vi "elliptsoid fitting.vi"(11 "data in":dbl[][](array[numeric])) -> (1 "b":dbl, 2 "n":dbl[](array[numeric]), 3 "M":T1)   [LabVIEW 2021]
uses:
  <vilib>/Analysis/Matrix/Datatypes/RealMatrix.ctl
  <vilib>/Analysis/7linalg.llb/Eigenvalue and Vectors Output Option.ctl
  <vilib>/Analysis/baseanly.llb/Real A x B.vi
  <vilib>/Analysis/_algsub.llb/Real PseudoInverse Matrix.vi
  <vilib>/Analysis/7linalg.llb/Real Transpose Matrix.vi
  <vilib>/Analysis/7linalg.llb/Real Generalized Eigenvalues and Vectors.vi
  <vilib>/Analysis/baseanly.llb/A x Vector.vi
  <vilib>/Analysis/Matrix/Numeric/Subtract/Subtract - RM,RM.vi
  <vilib>/Analysis/NI_AALBase.lvlib
  <vilib>/Analysis/NI_AALPro.lvlib
  <vilib>/Analysis/Matrix/NI_Matrix.lvlib
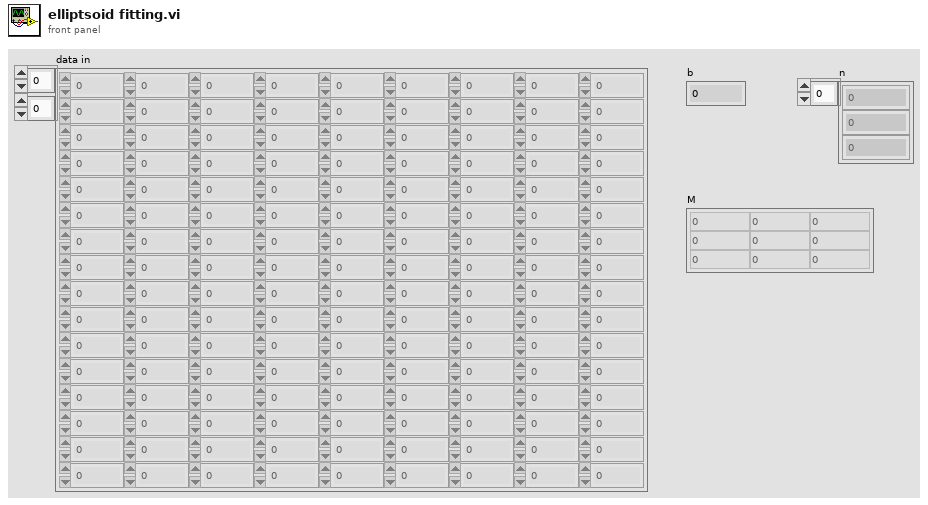
[diagram p1: front panel]
types:
  T1 = typedef "NI_Matrix.lvlib/RealMatrix.ctl" = dbl[][]
  T2 = typedef "NI_AALPro.lvlib/Eigenvalue and Vectors Output Option.ctl" = i32
  T3 = typedef "NI_Matrix.lvlib/ComplexMatrix.ctl" = cdb[][]
  T4 = cluster{"[0]":dbl, "[1]":dbl, "[2]":dbl, "[3]":dbl, "[4]":dbl, "[5]":dbl, "[6]":dbl, "[7]":dbl, "[8]":dbl, "[9]":dbl}
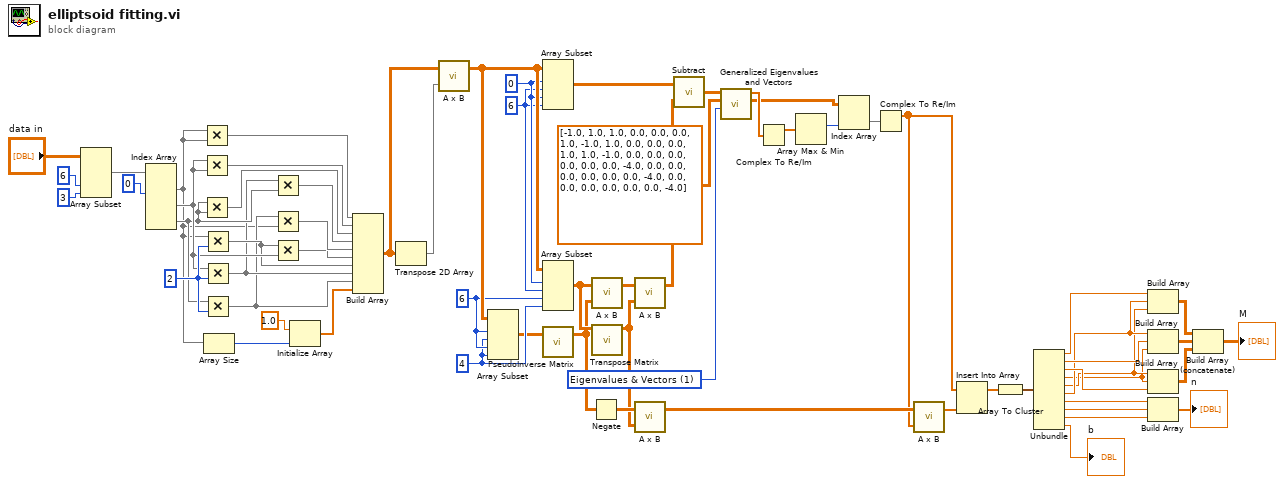
[diagram p0: block diagram]
diagram:
  w31 = T2 1 items=["Eigenvalues", "Eigenvalues & Vectors"] ("output option")
  w37 = 4 ("length")
  w38 = 6 ("index")
  w39 = 6 ("length")
  w40 = 0 ("index")
  w56 = 2 ("y")
  n1 = Array Subset(array="data in", index (col)=6 ("index"), length (col)=3 ("length")) -> (w61:dbl[][])  [unwired: 2 in]
  n2 = Index Array(array=w61, index (col) #1=0 ("disabled index (col)")) -> (element #1=w46:dbl[], element #2=w54:dbl[], element #3=w53:dbl[])  [unwired: 5 in]
  n3 = Multiply(x=w46, y=w46) -> (x*y=w59:dbl[])
  n4 = Multiply(x=w54, y=w54) -> (x*y=w58:dbl[])
  n5 = Multiply(x=w53, y=w53) -> (x*y=w57:dbl[])
  n6 = Multiply(x=w46, y=w56) -> (x*y=w50:dbl[])
  n7 = Multiply(x=w54, y=w56) -> (x*y=w49:dbl[])
  n8 = Multiply(x=w53, y=w56) -> (x*y=w48:dbl[])
  n9 = Array Size(array=w46) -> (size(s)=w45:i32)
  n10 = Multiply(x=w49, y=w53) -> (x*y=w55:dbl[])
  n11 = Multiply(x=w48, y=w46) -> (x*y=w52:dbl[])
  n12 = Multiply(x=w50, y=w54) -> (x*y=w51:dbl[])
  n13 = Initialize Array(1.0 ("element"), w45) -> (w44:dbl[])
  n14 = Build Array(w59, w58, w57, w55, w52, w51, w50, w49, w48, w44) -> (w43:dbl[][])
  n15 = Transpose 2D Array(2D array=w43) -> (transposed array=w42:dbl[][])
  n16 = call-poly <vilib>:"A x B.vi"("B"=w42, "A"=w43) -> ("A x B"=w41:T1)  [unwired: 1 out]
  n17 = Array Subset(array=w41, index (row)=w38, length (row)=w37, index (col)=w38, length (col)=w37) -> (w36:T1)
  n18 = Array Subset(array=w41, index (row)=w40, length (row)=w39, index (col)=w40, length (col)=w39) -> (w35:T1)
  n19 = Array Subset(array=w41, index (row)=w40, length (row)=w39, index (col)=w38, length (col)=w37) -> (w34:T1)
  n20 = call-poly <vilib>:"PseudoInverse Matrix.vi"("Input Matrix"=w36) -> ("PseudoInverse Matrix"=w24:T1)  [unwired: 1 in, 1 out]
  n21 = Negate(x=w24) -> (-x=w23:T1)
  n22 = call-poly <vilib>:"A x B.vi"("B"=w24, "A"=w34) -> ("A x B"=w33:T1)  [unwired: 1 out]
  n23 = call-poly <vilib>:"Transpose Matrix.vi"("Input Matrix"=w34) -> ("Matrix Transpose"=w22:T1)  [unwired: 9 in, 1 out]
  n24 = call-poly <vilib>:"A x B.vi"("B"=w22, "A"=w33) -> ("A x B"=w32:T1)  [unwired: 1 out]
  n25 = call-poly <vilib>:"A x B.vi"("B"=w22, "A"=w23) -> ("A x B"=w21:T1)  [unwired: 1 out]
  n26 = call-poly <vilib>:"Subtract.vi"("Real Matrix B"=w32, "Real Matrix A"=w35) -> ("A - B"=w29:T1)
  n27 = call-poly <vilib>:"Generalized Eigenvalues and Vectors.vi"("output option"=w31, "B"=dbl[][] [[-1.0, 1.0, 1.0, 0.0, 0.0, 0.0], [1.0, -1.0, 1.0, 0.0, 0.0, 0.0], [1.0, 1.0, -1.0, 0.0, 0.0, 0.0], [0.0, 0.0, 0.0, -4.0, 0.0, 0.0], [0.0, 0.0, 0.0, 0.0, -4.0, 0.0], [0.0, 0.0, 0.0, 0.0, 0.0, -4.0]], "A"=w29) -> ("Eigenvectors"=w26:T3, "Eigenvalues"=w28:cdb[])  [unwired: 3 in, 1 out]
  n28 = Complex To Re/Im(x + iy=w28) -> (x=w27:dbl[])  [unwired: 1 out]
  n29 = Array Max & Min(array=w27) -> (max index (indices)=w1:i32)  [unwired: 3 out]
  n30 = Index Array(array=w26, index (col)=w1) -> (element=w25:cdb[])  [unwired: 1 in]
  n31 = Complex To Re/Im(x + iy=w25) -> (x=w20:dbl[])  [unwired: 1 out]
  n32 = call-poly <vilib>:"A x B.vi"("Vector"=w20, "A"=w21) -> ("A x Vector"=w19:dbl[])  [unwired: 1 out]
  n33 = Insert Into Array(array=w20, new element=w19) -> (w18:dbl[])  [unwired: 1 in]
  n34 = Array To Cluster(array=w18) -> (cluster=w17:T4)
  n35 = Unbundle(w17) -> ("[0]"=w12:dbl, "[1]"=w11:dbl, "[2]"=w10:dbl, "[3]"=w7:dbl, "[4]"=w8:dbl, "[5]"=w9:dbl, "[6]"=w6:dbl, "[7]"=w5:dbl, "[8]"=w4:dbl, "[9]"=→"b":dbl)
  n36 = Build Array(w12, w9, w8) -> (w16:T1)
  n37 = Build Array(w9, w11, w7) -> (w15:T1)
  n38 = Build Array(w8, w7, w10) -> (w14:T1)
  n39 = Build Array(w6, w5, w4) -> (→"n":dbl[])
  n40 = Build Array (concatenate)(w16, w15, w14) -> (→"M":T1)
